vi "DELETEstartIVAndWait.vi"(8 "error in (no error)":errorcluster, 11 "Instrument.Lockin in":refnum<class "Instrument.Lockin.lvclass">) -> (0 "error out":errorcluster, 2 "AI Waveform":waveform(dbl)[](array[waveform]), 3 "Instrument.Lockin out":refnum<class "Instrument.Lockin.lvclass">)   [LabVIEW 2019, in "Instrument.Lockin.lvclass"]
uses:
  Instrument.Lockin.lvclass
panel:
  in  "stop":bool
  out "timer (s)":dbl=1.2239999771118164
  # "This VI triggers the lockin and waits until the acquisition is complete"
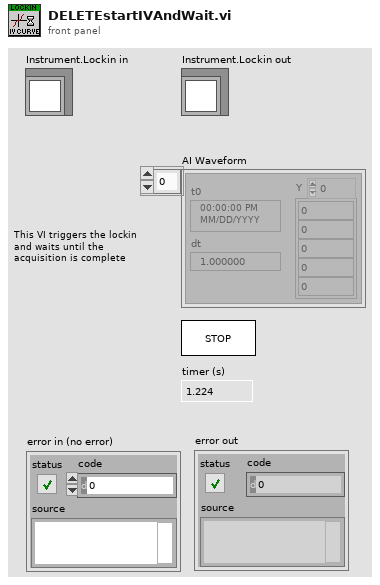
[diagram p1: front panel]
types:
  T1 = typedef "Instrument.DAQ.lvclass/AO.Channel--Cluster--Array.ctl" = T2[]
  T2 = typedef "Instrument.DAQ.lvclass/AO.Channel--Cluster.ctl" = cluster{"Enable?":bool, "Channel":i32, "Amplitude":dbl, "Offset":dbl, "Frequency":dbl, "Phase":dbl, "Function":T3, "Sweeping?":bool}
  T3 = typedef "Instrument.DAQ.lvclass/AO.Channel.Function--Enum.ctl" = enum16{"Sine", "Triangle", "Square"}
  T4 = typedef "Instrument.LockinAPI.lvclass/LockinAPI.getState.states--enum.ctl" = enum16{"idle", "created", "started", "stopped", "sweeping"}
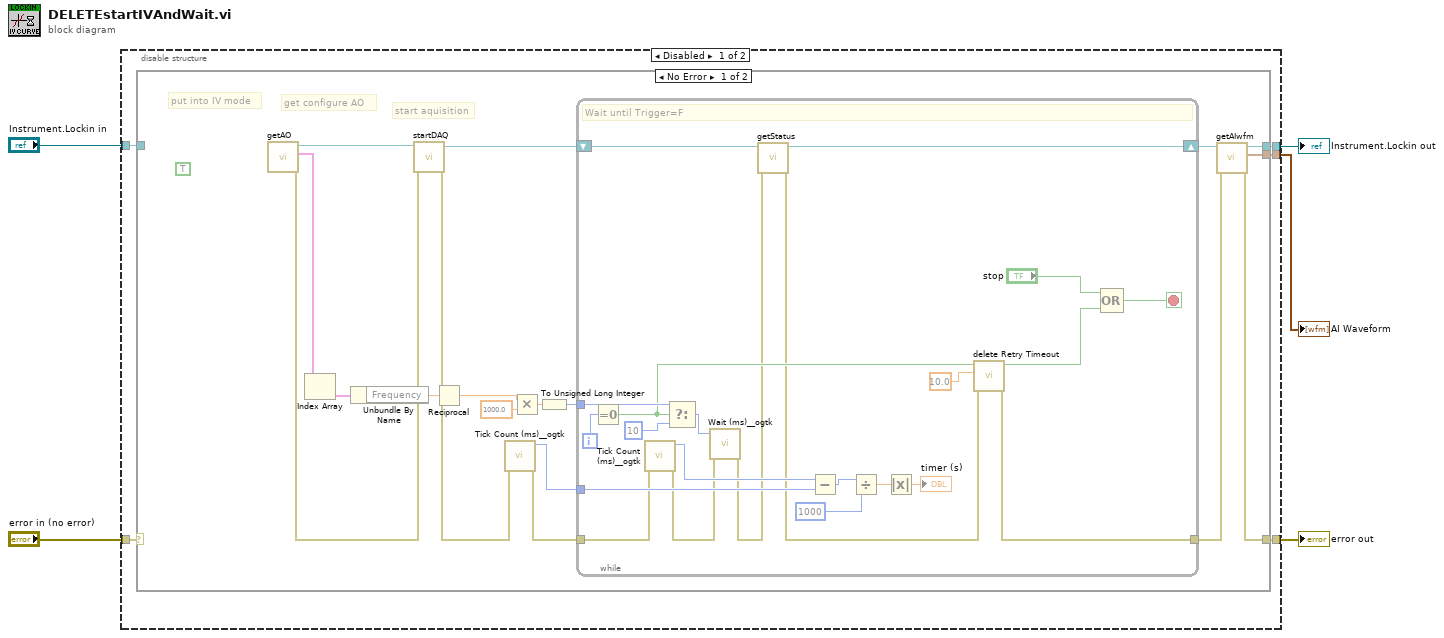
[diagram p0: block diagram]
diagram:
  n1 = disable-structure shown="Disabled" {
    disable-tunnel: [w10 _] -> w5
    disable-tunnel: [w9 _] -> w4
    disable-tunnel: "Instrument.Lockin in" -> [w8 _]
    disable-tunnel: [w7 _] -> w2
    disable-tunnel: "error in (no error)" -> [w6 _]
    frame Disabled {
      n2 = case shown="No Error" w6 {
        selector: w6 -> [w17 w58]
        tunnel: [w14 w58] -> w10
        tunnel: [w27 _] -> w9
        tunnel: w8 -> [w18 w57]
        tunnel: [w19 w57] -> w7
        frame No Error {
          (unwired) TRUE ("IV mode")
          # "start aquisition"
          # "get configure AO"
          # "put into IV mode"
          n3 = call-dynamic "getAO.vi"() -> ("error out"=w22:errorcluster, "AOconfig"=w13:T1, "Instrument.Lockin out"=w21:refnum<class "Instrument.Lockin.lvclass">, "error in (no error)"=w24:errorcluster, "Instrument.Lockin in"=w23:refnum<class "Instrument.Lockin.lvclass">)  [unwired: 7 in]
          n4 = Index Array(array=w13) -> (element=w12:T2)  [unwired: 1 in]
          n5 = Unbundle By Name(w12) -> ("Frequency"=w11:dbl)
          n6 = call-dynamic "startDAQ.vi"("error in (no error)"=w22, "Instrument.Lockin in"=w21) -> ("error out"=w20:errorcluster, "Instrument.Lockin out"=w25:refnum<class "Instrument.Lockin.lvclass">)  [unwired: 8 in]
          n7 = Reciprocal(x=w11) -> (1/x=w29:dbl)
          n8 = call <userlib>:"Tick Count (ms)__ogtk.vi"("error in (no error)"=w20) -> ("error out"=w16:errorcluster, "millisecond timer value"=w32:u32)  [unwired: 9 in]
          n9 = Multiply(x=w29, y=1000.0) -> (x*y=w30:dbl)
          n10 = To Unsigned Long Integer(number=w30) -> (unsigned 32bit integer=w28:u32)
          n11 = while {
            tunnel: w32 -> [w54]
            tunnel: w28 -> [w49]
            tunnel: w16 -> [w40]
            tunnel: [w39] -> w15
            shift-right: [w47] -> w26
            shift-left: w25 -> [w46]
            i -> [w51]
            stop <- w53 stop-if-true
            # "Wait until Trigger=F"
            n12 = Equal To 0?(x=w51) -> (x = 0?=w42:bool)
            n13 = call <userlib>:"Tick Count (ms)__ogtk.vi"("error in (no error)"=w40) -> ("error out"=w52:errorcluster, "millisecond timer value"=w55:u32)  [unwired: 9 in]
            n14 = Select(t=w49, s=w42, f=u32 10) -> (s? t:f=w50:u32)
            n15 = call <userlib>:"Wait (ms)__ogtk.vi"("error in (no error)"=w52, "milliseconds to wait"=w50) -> ("error out"=w37:errorcluster)  [unwired: 8 in, 1 out]
            n16 = call-dynamic "getStatus.vi"("error in (no error)"=w37, "Instrument.Lockin"=w46) -> ("error out"=w38:errorcluster, "state"=w48:T4, "Instrument.Lockin"=w47:refnum<class "Instrument.Lockin.lvclass">)  [unwired: 7 in]
            n17 = Subtract(x=w55, y=w54) -> (x-y=w43:u32)
            n18 = Divide(x=w43, y=u32 1000 ("x")) -> (x/y=w45:dbl)
            n19 = Absolute Value(x=w45) -> (abs(x)=→"timer (s)":dbl)
            n20 = call "delete Retry Timeout.vi"("error in (no error)"=w38, "time (s) [10 s]"=10.0, "reset"=w42) -> ("error out"=w39:errorcluster, "Timeout?"=w34:bool)  [unwired: 7 in]
            n21 = Compound Arithmetic op=OR("stop", w34) -> (w53:bool, w36:bool)
          }
          n22 = call-dynamic "getAIwfm.vi"("error in (no error)"=w15, "Instrument.Lockin in"=w26) -> ("error out"=w14:errorcluster, "AI Waveform"=w27:waveform(dbl)[], "Instrument.Lockin out"=w19:refnum<class "Instrument.Lockin.lvclass">)  [unwired: 7 in]
        }
        frame Error {
        }
      }
    }
    frame Enabled {
    }
  }
  "error out" <- w5
  "AI Waveform" <- w4
  "Instrument.Lockin out" <- w2
